vi "Open.vi"(8 "error in (no error)":errorcluster, 10 "I2C Channel":u8, 11 "I2C in":refnum<class "I2C.lvclass">) -> (0 "error out":errorcluster, 3 "I2C out":refnum<class "I2C.lvclass">)   [LabVIEW 2014, in "I2C.lvclass"]
doc: "Open the specified I2C channel. If the device has a single I2C master it is channel 0. If the device has more than one I2C master the logical first I2C master is channel 0, the next is channel 1, etc."
uses:
  I2C.lvclass
  I2C.lvclass/I2C.ctl
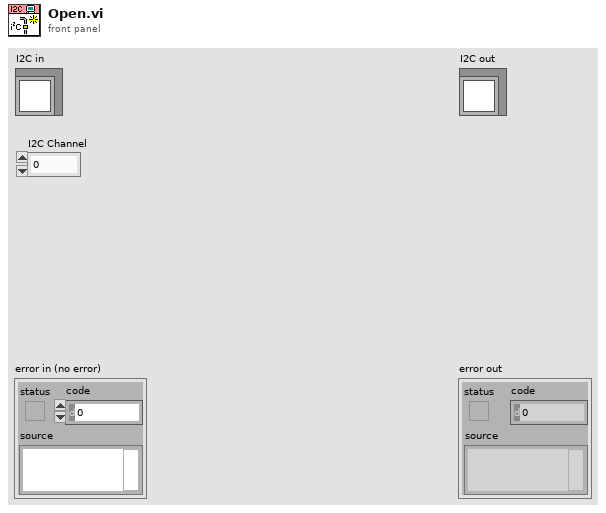
[diagram p1: front panel]
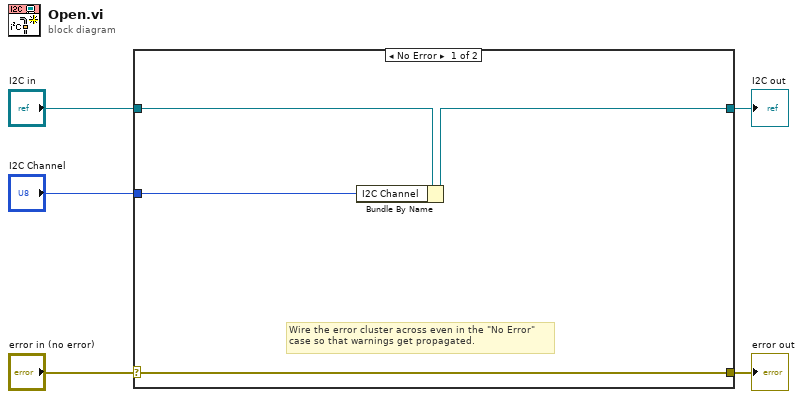
[diagram p0: block diagram]
diagram:
  n1 = case shown="No Error" "error in (no error)" {
    selector: "error in (no error)" -> [w8 w11]
    tunnel: [w8 w11] -> w4
    tunnel: [w7 w10] -> w2
    tunnel: "I2C in" -> [w9 w10]
    tunnel: "I2C Channel" -> [w6 _]
    frame No Error {
      # "Wire the error cluster across even in the \"No Error\"\ncase so that warnings get propagated."
      n2 = Bundle By Name(cluster=w9, "I2C Channel"=w6) -> (w7:refnum<class "I2C.lvclass">)
    }
    frame Error {
    }
  }
  "error out" <- w4
  "I2C out" <- w2
